vi "get_Register_Offset.vi"(8 "error in (no error)":errorcluster, 10 "session":u32, 11 "Name":string) -> (0 "error out":errorcluster, 1 "RegisterOffset":u32, 2 "Register Name":string, 3 "session out":u32)   [LabVIEW 2021, in "FPGA Addon Engine.lvlib"]
uses:
  Types/Register Settings.ctl
  Addon Shared/Types/FPGA Addon Data Type.ctl
  Addon Shared/Types/Scalar Type.ctl
  FPGA Addon Engine.lvlib
  Addon Shared/FPGA Addon Shared.lvlib
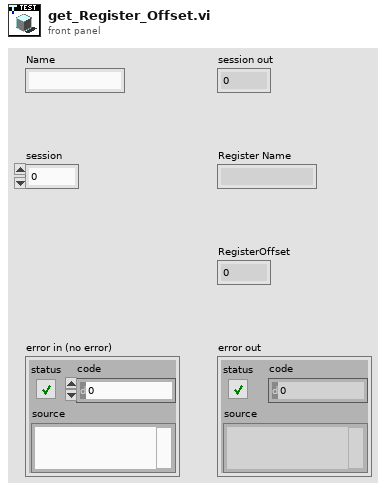
[diagram p1: front panel]
types:
  T1 = typedef "FPGA Addon Engine.lvlib/Register Settings.ctl" = cluster{"Name":string, "Data Type":T2, "session":u32, "Scalar Type":T3, "Index":i32, "Length":i32, "attributes":variant, "default value":variant, "RegisterOffset":u32}
  T2 = typedef "FPGA Addon Shared.lvlib/FPGA Addon Data Type.ctl" = enum8{"<Null>", "I8", "I16", "I32", "I64", "U8", "U16", "U32", "U64", "SGL", "Boolean", "Analog PWM In Settings", "Analog PWM In", "Digital PWM In Settings", "Digital PWM In", "Digital PWM Out", "Sine Out", "FXP", "FXP+/-24.5", "FXP+/-16.5", "FXP+/-32.8", "FXP+/-64.32", "FXP+/-16.7", "FXP+/-20.5", "FXP+/-27.5", "FXP+/-32.16", "FXP+16.3", "FXP+18.3", "Digital Static In", "Digital Static Out", "Digital Static In Settings", "Digital WSS Out", "Quad Encoder Settings", "Quad Encoder In", "Group"}
  T3 = typedef "FPGA Addon Shared.lvlib/Scalar Type.ctl" = enum16{"Standard", "Bitpacked"}
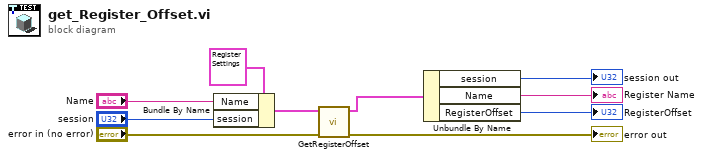
[diagram p0: block diagram]
diagram:
  n1 = Bundle By Name(cluster=T1 {"Name"="", "Data Type"=enum."<Null>", "session"=0, "Scalar Type"=enum."Standard", "Index"=0, "Length"=0, "attributes"=variant, "default value"=variant, "RegisterOffset"=0} ("element in"), "Name"="Name", "session"="session") -> (w9:T1)
  n2 = call "GetRegisterOffset.vi"("error in (no error)"="error in (no error)", "element in"=w9) -> ("error out"=→"error out":errorcluster, "element out"=w4:T1)  [unwired: 7 in, 1 out]
  n3 = Unbundle By Name(w4) -> ("session"=→"session out":u32, "Name"=→"Register Name":string, "RegisterOffset"=→"RegisterOffset":u32)
